vi "Update coins.vi"(8 "error in (no error)":errorcluster, 10 "Coins":cluster{"1":bool, "2":bool, "5":bool, "10":bool}, 11 "Quetzal Actor in":refnum<class "Quetzal Actor.lvclass">) -> (0 "error out":errorcluster, 3 "Quetzal Actor out":refnum<class "Quetzal Actor.lvclass">)   [LabVIEW 2020, in "Quetzal Actor.lvlib" / "Quetzal Actor.lvclass"]
uses:
  Quetzal Actor.lvclass
  C:/Program Files/National Instruments/LabVIEW 2020/vi.lib/ActorFramework/Actor/Actor.lvclass
  <vilib>/ActorFramework/Actor/Actor.lvclass/Actor.ctl
  Quetzal Actor.lvclass/Quetzal Actor.ctl
  UI Actor Messages/Credit update Msg/Credit update Msg.lvclass/Credit update Msg.ctl
  <vilib>/ActorFramework/Message Enqueuer/Message Enqueuer.lvclass/Message Enqueuer.ctl
  <vilib>/ActorFramework/Message Enqueuer/Enqueue.vi
  UI Actor Messages/Credit update Msg/Credit update Msg.lvclass
  C:/Program Files/National Instruments/LabVIEW 2020/vi.lib/ActorFramework/Message/Message.lvclass
  <vilib>/ActorFramework/Message Priority Queue/Priority Enqueue.vi
  <vilib>/ActorFramework/Actor/Actor.lvclass
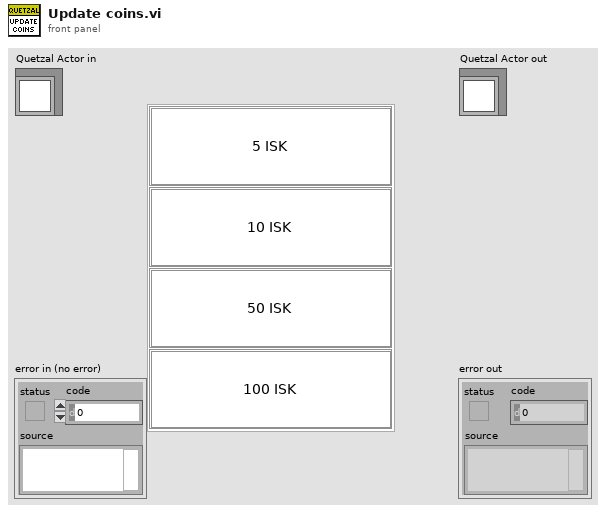
[diagram p1: front panel]
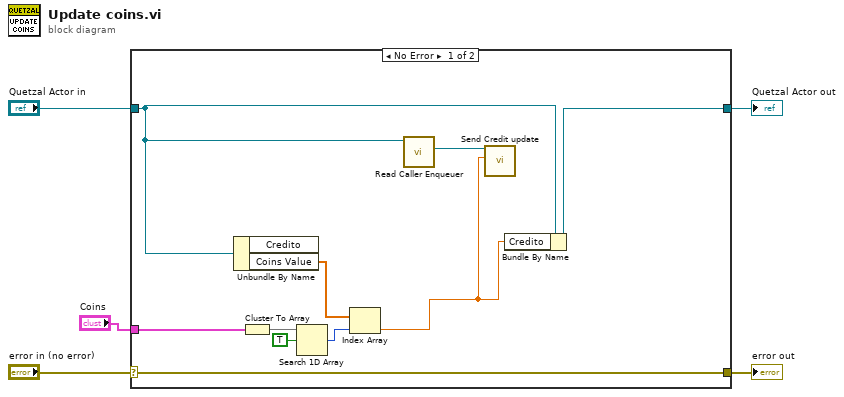
[diagram p0: block diagram]
diagram:
  n1 = case shown="No Error" "error in (no error)" {
    selector: "error in (no error)" -> [w15 w17]
    tunnel: [w15 w17] -> w4
    tunnel: [w8 w16] -> w2
    tunnel: "Quetzal Actor in" -> [w9 w16]
    tunnel: "Coins" -> [w7 _]
    frame No Error {
      n2 = Unbundle By Name(w9) -> ("Coins Value"=w11:dbl[])  [unwired: 1 out]
      n3 = Cluster To Array(cluster=w7) -> (array=w14:bool[])
      n4 = Search 1D Array(1D array=w14, element=TRUE) -> (index of element=w12:i32)  [unwired: 1 in]
      n5 = Index Array(array=w11, index=w12) -> (element=w6:dbl)
      n6 = call <vilib>:"Read Caller Enqueuer.vi"("Actor"=w9) -> ("Caller Enqueuer"=w10:refnum<class "Message Enqueuer.lvclass">)  [unwired: 10 in]
      n7 = call "Send Credit update.vi"("Creditp"=w6, "Message Enqueuer"=w10) -> ()  [unwired: 8 in, 2 out]
      n8 = Bundle By Name(cluster=w9, "Credito"=w6) -> (w8:refnum<class "Quetzal Actor.lvclass">)
    }
    frame Error {
    }
  }
  "error out" <- w4
  "Quetzal Actor out" <- w2
